vi "enhanc_factor_2024.vi"(2 "saturated vapor pressure [Pa]":dbl=2339.25, 3 "Temperature / K":dbl=293.15 format="%#_13g", 4 "Pressure / Pa":dbl=101325.0 format="%#_13g") -> (0 "psat/p > 1/fe !":bool, 1 "enhancement factor":dbl=1.0283727476805382 format="%.5f")   [LabVIEW 2016]
uses:
  <vilib>/Analysis/NI_AALPro.lvlib
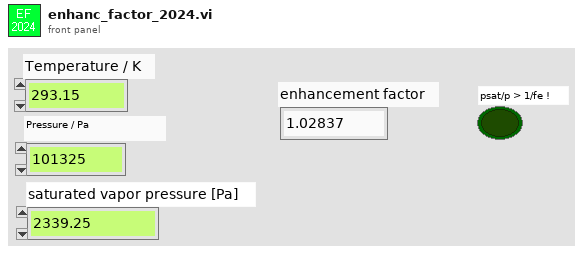
[diagram p1: front panel]
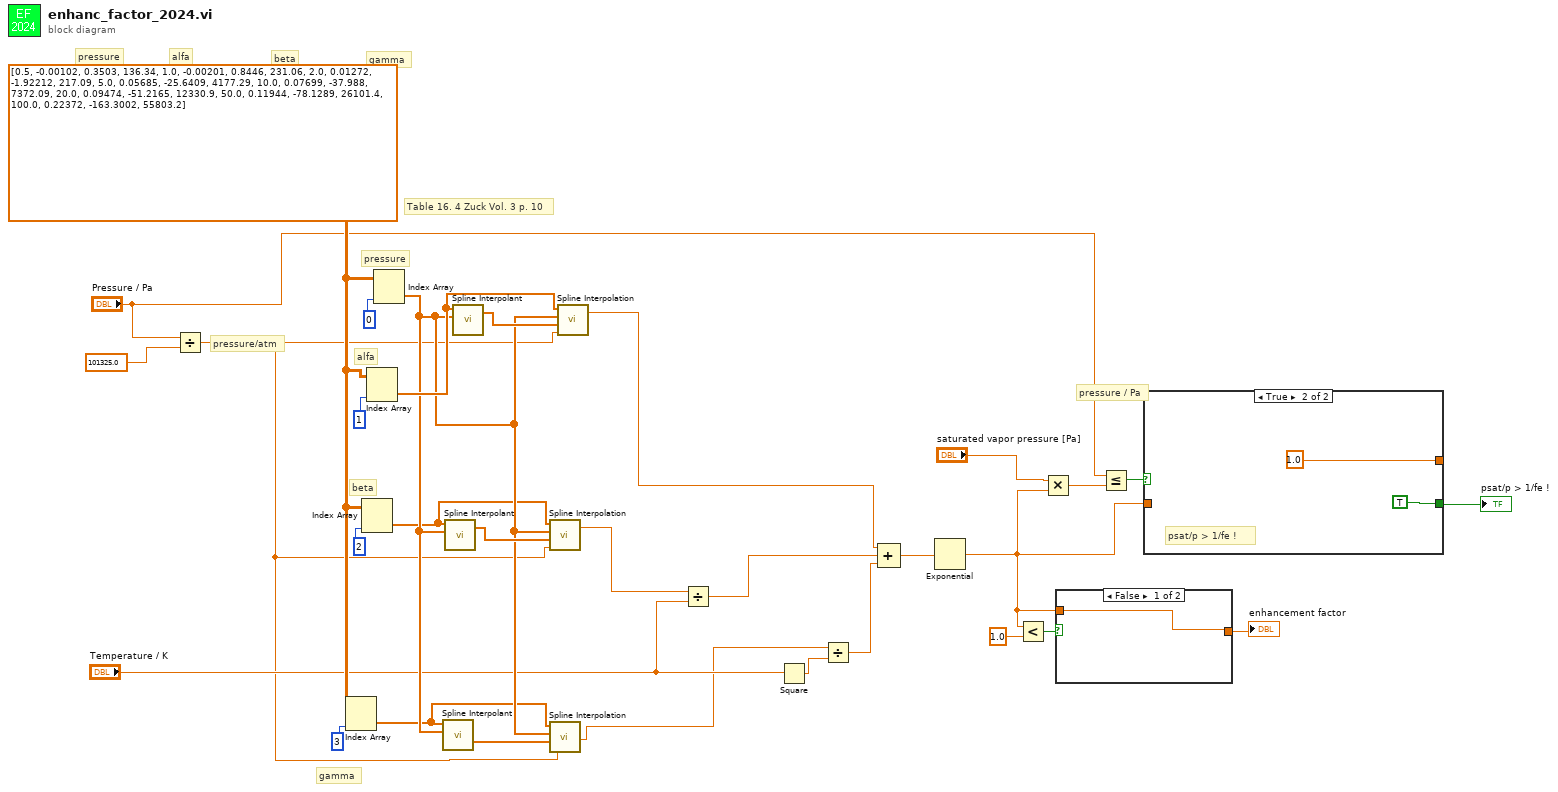
[diagram p0: block diagram]
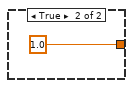
[diagram p2: hidden frame]
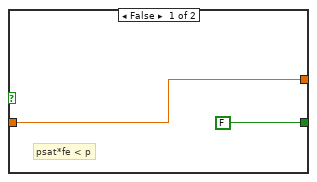
[diagram p3: hidden frame]
diagram:
  w24 = dbl[][] [[0.5, -0.00102, 0.3503, 136.34], [1.0, -0.00201, 0.8446, 231.06], [2.0, 0.01272, -1.92212, 217.09], [5.0, 0.05685, -25.6409, 4177.29], [10.0, 0.07699, -37.988, 7372.09], [20.0, 0.09474, -51.2165, 12330.9], [50.0, 0.11944, -78.1289, 26101.4], [100.0, 0.22372, -163.3002, 55803.2]]
  # "pressure / Pa"
  # "Table 16. 4 Zuck Vol. 3 p. 10"
  # "pressure/atm"
  # "gamma"
  # "beta"
  # "alfa"
  # "pressure"
  # "gamma"
  # "beta"
  # "alfa"
  # "pressure"
  n1 = Divide(x="Pressure / Pa", y=101325.0) -> (x/y=w10:dbl)
  n2 = Index Array(array=w24, index (col)=3 ("index (row)")) -> (element=w20:dbl[])  [unwired: 1 in]
  n3 = Index Array(array=w24, index (col)=2 ("index (row)")) -> (element=w21:dbl[])  [unwired: 1 in]
  n4 = Index Array(array=w24, index (col)=1 ("index (row)")) -> (element=w23:dbl[])  [unwired: 1 in]
  n5 = Index Array(array=w24, index (col)=0 ("index (row)")) -> (element=w22:dbl[])  [unwired: 1 in]
  n6 = call <vilib>:"Spline Interpolant.vi"("X"=w22, "Y"=w20) -> ("Interpolant"=w25:dbl[])  [unwired: 2 in, 1 out]
  n7 = call <vilib>:"Spline Interpolant.vi"("X"=w22, "Y"=w21) -> ("Interpolant"=w27:dbl[])  [unwired: 2 in, 1 out]
  n8 = call <vilib>:"Spline Interpolant.vi"("X"=w22, "Y"=w23) -> ("Interpolant"=w29:dbl[])  [unwired: 2 in, 1 out]
  n9 = call <vilib>:"Spline Interpolation.vi"("x value"=w10, "Interpolant"=w27, "X"=w22, "Y"=w21) -> ("interpolation value"=w15:dbl)  [unwired: 1 out]
  n10 = call <vilib>:"Spline Interpolation.vi"("x value"=w10, "Interpolant"=w25, "X"=w22, "Y"=w20) -> ("interpolation value"=w12:dbl)  [unwired: 1 out]
  n11 = call <vilib>:"Spline Interpolation.vi"("x value"=w10, "Interpolant"=w29, "X"=w22, "Y"=w23) -> ("interpolation value"=w16:dbl)  [unwired: 1 out]
  n12 = Divide(x=w15, y="Temperature / K") -> (x/y=w14:dbl)
  n13 = Square(x="Temperature / K") -> (x^2=w19:dbl)
  n14 = Divide(x=w12, y=w19) -> (x/y=w13:dbl)
  n15 = Compound Arithmetic op=ADD(w16, w14, w13) -> (w18:dbl)
  n16 = Exponential(1:w18) -> (0:w2:dbl)
  n17 = Less?(x=w2, y=1.0) -> (x < y?=w3:bool)
  n18 = Multiply(x="saturated vapor pressure [Pa]", y=w2) -> (x*y=w9:dbl)
  n19 = case shown="False" w3 {
    tunnel: [w32 1.0] -> w1
    tunnel: w2 -> [w32 _]
    frame False {
    }
    frame True {
    }
  }
  "enhancement factor" <- w1
  n20 = Less Or Equal?(x="Pressure / Pa", y=w9) -> (x <= y?=w8:bool)
  n21 = case shown="True" w8 {
    tunnel: w2 -> [w35 _]
    tunnel: [w35 1.0] -> _
    tunnel: [FALSE TRUE] -> w5
    frame False {
      # "psat*fe < p"
    }
    frame True {
      # "psat/p > 1/fe !"
    }
  }
  "psat/p > 1/fe !" <- w5
